vi "Dashboard Main.vi"() -> ()   [LabVIEW 2016]
uses:
  <vilib>/event_ctls.llb/eventvkey.ctl
  <vilib>/Rock Robotics/WPI/Dashboard/WPI_DashboardLogging Global.vi
  <vilib>/Utility/miscctls.llb/LVRowAndColumnTypeDef.ctl
  <vilib>/Rock Robotics/Network Tables/NT Read Numeric Array.vi
  <vilib>/Rock Robotics/Network Tables/NT Read Boolean.vi
panel:
  out "Gear State":string
  in  "Camera Name 2":string(combo)="No Camera Selection"
  in  "Camera Settings Right":T1={"Frame Rate"=30, "Compression"=30, "Size"=1, "DB Camera Config"=FALSE} {"Frame Rate" scale=1.0..30.0; "Compression" scale=100.0..-1.0; "Size" items=["640x480", "320x240", "160x120"]}
  in  "Camera Name Right":string(combo)="No Camera Selection"
  out "Camera Info":cluster{"Mbps LED":bool, "Mbps":dbl, "fps":dbl} {"fps" format="%#.1g"; "Mbps" format="%#.1g"}
  in  "Camera Settings":T1={"Frame Rate"=30, "Compression"=30, "Size"=1, "DB Camera Config"=FALSE} {"Frame Rate" scale=1.0..30.0; "Compression" scale=100.0..-1.0; "Size" items=["640x480", "320x240", "160x120"]}
  in  "TCP":refnum<k5>
  in  "Rec Mode":enum32{"Stop", "Record", "Playback"}(radio)
  out "Robot IP":string
  out "Image Message":string="Timeout in Camera Communications"
  in  "Dashboard Tab":T2(tab)
  in  "Select Auto":string(combo)="Select Autonomous ..."
  out "NT Connection":bool
  out "MotorChart R":cluster{"Numeric":dbl, "Numeric":dbl}(graph)
  out "MotorChart L":cluster{"Numeric":dbl, "Numeric":dbl}(graph)
  out "MotorSliders R":cluster{"MotorSlide1":dbl, "MotorSlide2":dbl} {"MotorSlide2" scale=-1.0..1.0 scale format="%#_2e"; "MotorSlide1" scale=-1.0..1.0 scale format="%#_2e"}
  out "MotorSliders L":cluster{"MotorSlide1":dbl, "MotorSlide2":dbl} {"MotorSlide2" scale=-1.0..1.0 scale format="%#_2e"; "MotorSlide1" scale=-1.0..1.0 scale format="%#_2e"}
  out "Gyro":dbl(knob) scale=0.0..360.0
  out "JS1 Z":dbl(slide) scale=-1.0..1.0 scale format="%#_2e"
  out "JS1 Graph":cluster{"X":dbl, "Y":dbl}[](graph)
  out "JS1 Buttons":T3
  out "JS2 Z":dbl(slide) scale=-1.0..1.0 scale format="%#_2e"
  out "JS2 Graph":cluster{"X":dbl, "Y":dbl}[](graph)
  out "JS2 Buttons":T3
  out "Mode":T4(ring)=enum."Auto Disabled"
  out "Camera Image Right":T5(plugin-control)
  in  "Test Slider":dbl(slide) scale=0.0..100.0 scale format="%#_3g"
  in  "On/Off":bool caption="Solenoid"
  in  "Test Name":u16(ring) items=["Select the test to run..."]
  in  "Test Tree":string(tree)
  in  "Motor":cluster{"Value":dbl, "Enable":bool} {"Value" scale=-1.0..1.0 scale format="%#_3g"}
  out "Progress":T6 {"Test Progress" scale=0.0..100.0}
  in  "Rev/Fwd":cluster{"Forward":bool, "Reverse":bool}
  in  "Test Ring":u16(ring) items=["Monochrome", "Color"]
  out "Cmd Status":string
  in  "Execute Command":bool
  in  "Command Params":string[][](table)
  in  "Command Selection":i32(listbox)
  in  "CheckList":i32(listbox)
  out "Tree":string(tree)
  out "Camera Image":T5(plugin-control)
  out "Background":bool
  in  "Camera Name":string(combo)="No Camera Selection"
  # "HW"
  # "HW"
  # "Joysticks"
  # "Drive Motors"
  # "Front"
  # "Right"
  # "Left"
  # "Back"
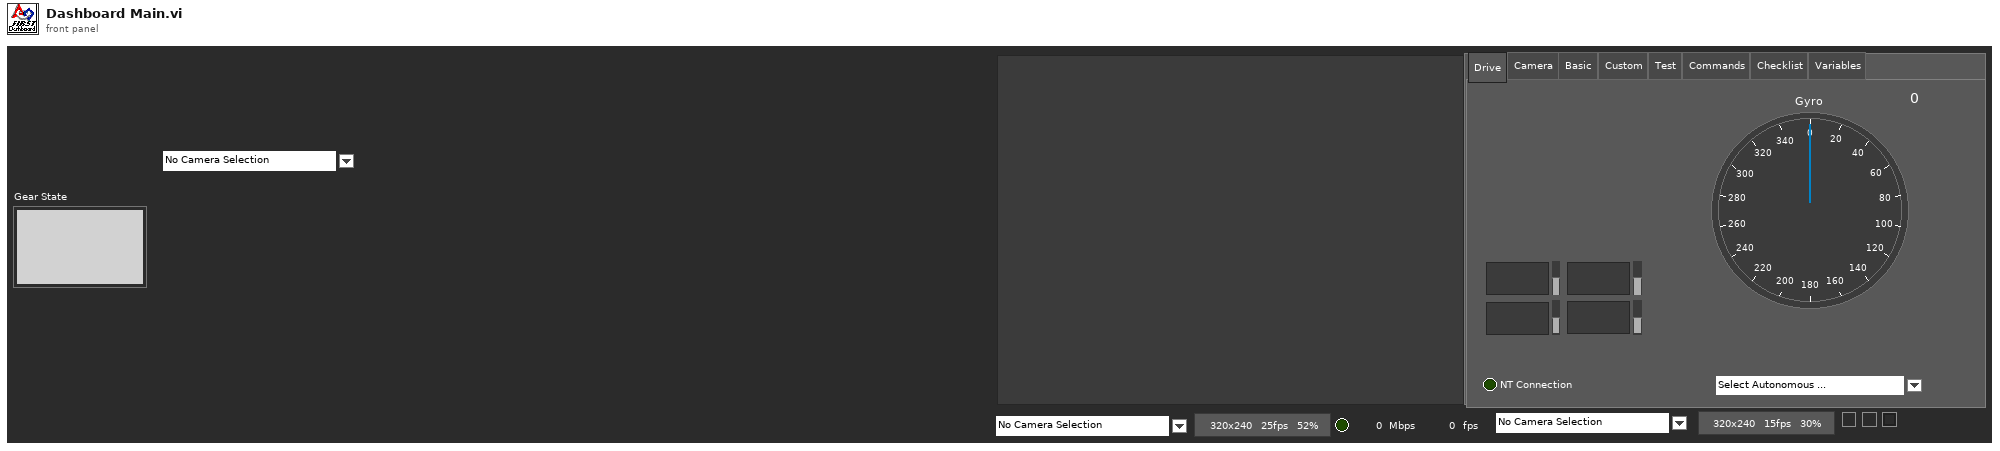
[diagram p1: front panel]
types:
  T1 = cluster{"Frame Rate":i32, "Compression":i32, "Size":u16, "DB Camera Config":bool}
  T2 = enum32{"Drive", "Camera", "Basic", "Custom", "Test", "Commands", "Checklist", "Variables"}
  T3 = cluster{bool, bool, bool, bool, bool, bool, bool, bool, bool, bool, bool, bool}
  T4 = enum8{"Tele-Op Disabled", "Tele-Op Enabled", "Auto Disabled", "Auto Enabled", "Test Disabled", "Test Enabled", "Disconnected", "No Code", "E-Stop"}
  T5 = typedef "IMAQ Image.ctl" = refnum<image>
  T6 = cluster{"Test Progress":u8, "Test Progress Text":string}
  T7 = typedef "Image Type" = u32
  T8 = cluster{"IDs":cluster{"RPC field ID":u16, "Unique ID":u16}, "String":string}
  T9 = enum32{"Drive", "Basic", "Custom", "Test", "Checklist", "Variables"}
  T10 = cluster{"Error Strings":string, "Disable Counts":cluster{u16, u16}, "Rail Faults":cluster{u16, u16, u16}, "Robot IP":string, "DB Mode":u8, "Event Info":cluster{"Name":string, "Type":u8, "Number":u16, "Replay":u8}}
  T11 = cluster{"Storage":cluster{"Disk Free":u64, "RAM Block":u32, "RAM free":u32}, "CPU Utilization":cluster{"CPU % ISR":sgl, "CPU % Time Crit":sgl, "CPU % Timed Str":sgl, "CPU % High":sgl, "CPU % Above":sgl, "CPU % Normal":sgl, "CPU % Low":sgl}, "CAN":cluster{"% Bus Utilization":sgl, "Bus Off Cnt":u32, "TX_FIFO Full Cnt":u32, "Receive Error Cnt":u8, "Transmit Error Cnt":u8}, "HID":cluster{"HID Outputs":u32, "Rumble Low":u16, "Rumble High":u16}[]}
  T12 = cluster{"Status bits":cluster{"Test Mode":bool, "Autonomous":bool, "Enabled":bool, "Code Start":bool, "Brownout":bool, "Reserved 2":bool, "Reserved 3":bool, "E-Stop":bool}, "Code Trace":cluster{"Disabled":bool, "TeleOp":bool, "Auto":bool, "Test":bool}, "Controller Type":enum16{"unknown", "cRIO", "roboRio"}, "Code?":enum16{"unknown", "noCode", "code"}, "Battery V":dbl}
  T13 = cluster{"Control Bits":cluster{"TestMode":bool, "Autonomous":bool, "Enabled":bool, "FMS Present":bool, bool, bool, bool, "E-Stop":bool}, "Team Station ":u8, "Countdown":sgl, "Joystick Values":cluster{"Axes":dbl[], "Buttons":bool[], "POVs":i16[]}[]}
  T14 = cluster{"Axes":dbl[], "Buttons":bool[], "POVs":i16[]}[]
  T15 = cluster{"Axes":dbl[], "Buttons":bool[], "POVs":i16[]}
  T16 = cluster{"Buttons[0]":bool, "Buttons[1]":bool, "Buttons[2]":bool, "Buttons[3]":bool, "Buttons[4]":bool, "Buttons[5]":bool, "Buttons[6]":bool, "Buttons[7]":bool, "Buttons[8]":bool, "Buttons[9]":bool, "Buttons[10]":bool, "Buttons[11]":bool}
  T17 = cluster{"Camera Image":refnum<vi>, "Dashboard Tab":refnum<vi>, "Background":refnum<vi>, "Rec Mode":refnum<vi>, "Test Slider":refnum<vi>, "On/Off ":refnum<vi>, "Test Ring":refnum<vi>, "Rev/Fwd":refnum<vi>, "Test Name":refnum<vi>, "Motor":refnum<vi>, "Progress":refnum<vi>, "CheckList":refnum<vi>, "Tree":refnum<vi>, "Test Tree":refnum<vi>, "Command Params":refnum<vi>, "Command Selection":refnum<vi>, "Execute Command":refnum<vi>, "Cmd Status":refnum<vi>, "Camera Settings":refnum<vi>, "Camera Name":refnum<vi>, "Camera Info":refnum<vi>, "Camera Settings Right":refnum<vi>, "Camera Name Right":refnum<vi>, "Camera Image Right":refnum<vi>}
  T18 = cluster{"Operation":enum16{"Update", "Clear"}, "Color Box":u32}[]
  T19 = typedef "eventvkey.ctl" = enum16{"ASCII", "Enter", "Return", "Shift", "Ctrl", "Alt", "Cmd", "Opt", "Caps", "NumLock", "Clear", "Break", "Up", "Down", "Left", "Right", "Insert", "Delete", "Home", "End", "PageUp", "PageDown", "Escape", "Help", "Pause", "ScrollLock", "F1", "F2", "F3", "F4", "F5", "F6", "F7", "F8", "F9", "F10", "F11", "F12", "F13", "F14", "F15", "F16", "F17", "F18", "F19", "F20", "F21", "F22", "F23", "F24", "Play", "VolumeUp", "VolumeDown", "Mute", "Two Byte Char"}
  T20 = cluster{"Image Size":bool, "Image Type":bool, "Pixel Value":bool, "ROI Information":bool, "Zoom Factor":bool}
  T21 = cluster{"Operation":enum16{"Update", "Clear"}, "Color Box":u32}
  T22 = typedef "LVRowAndColumnTypeDef.ctl" = cluster{"Row":i32, "Column":i32}
  T23 = cluster{"Shift":bool, "Ctrl":bool, "Alt":bool, "Cmd":bool, "Opt":bool}
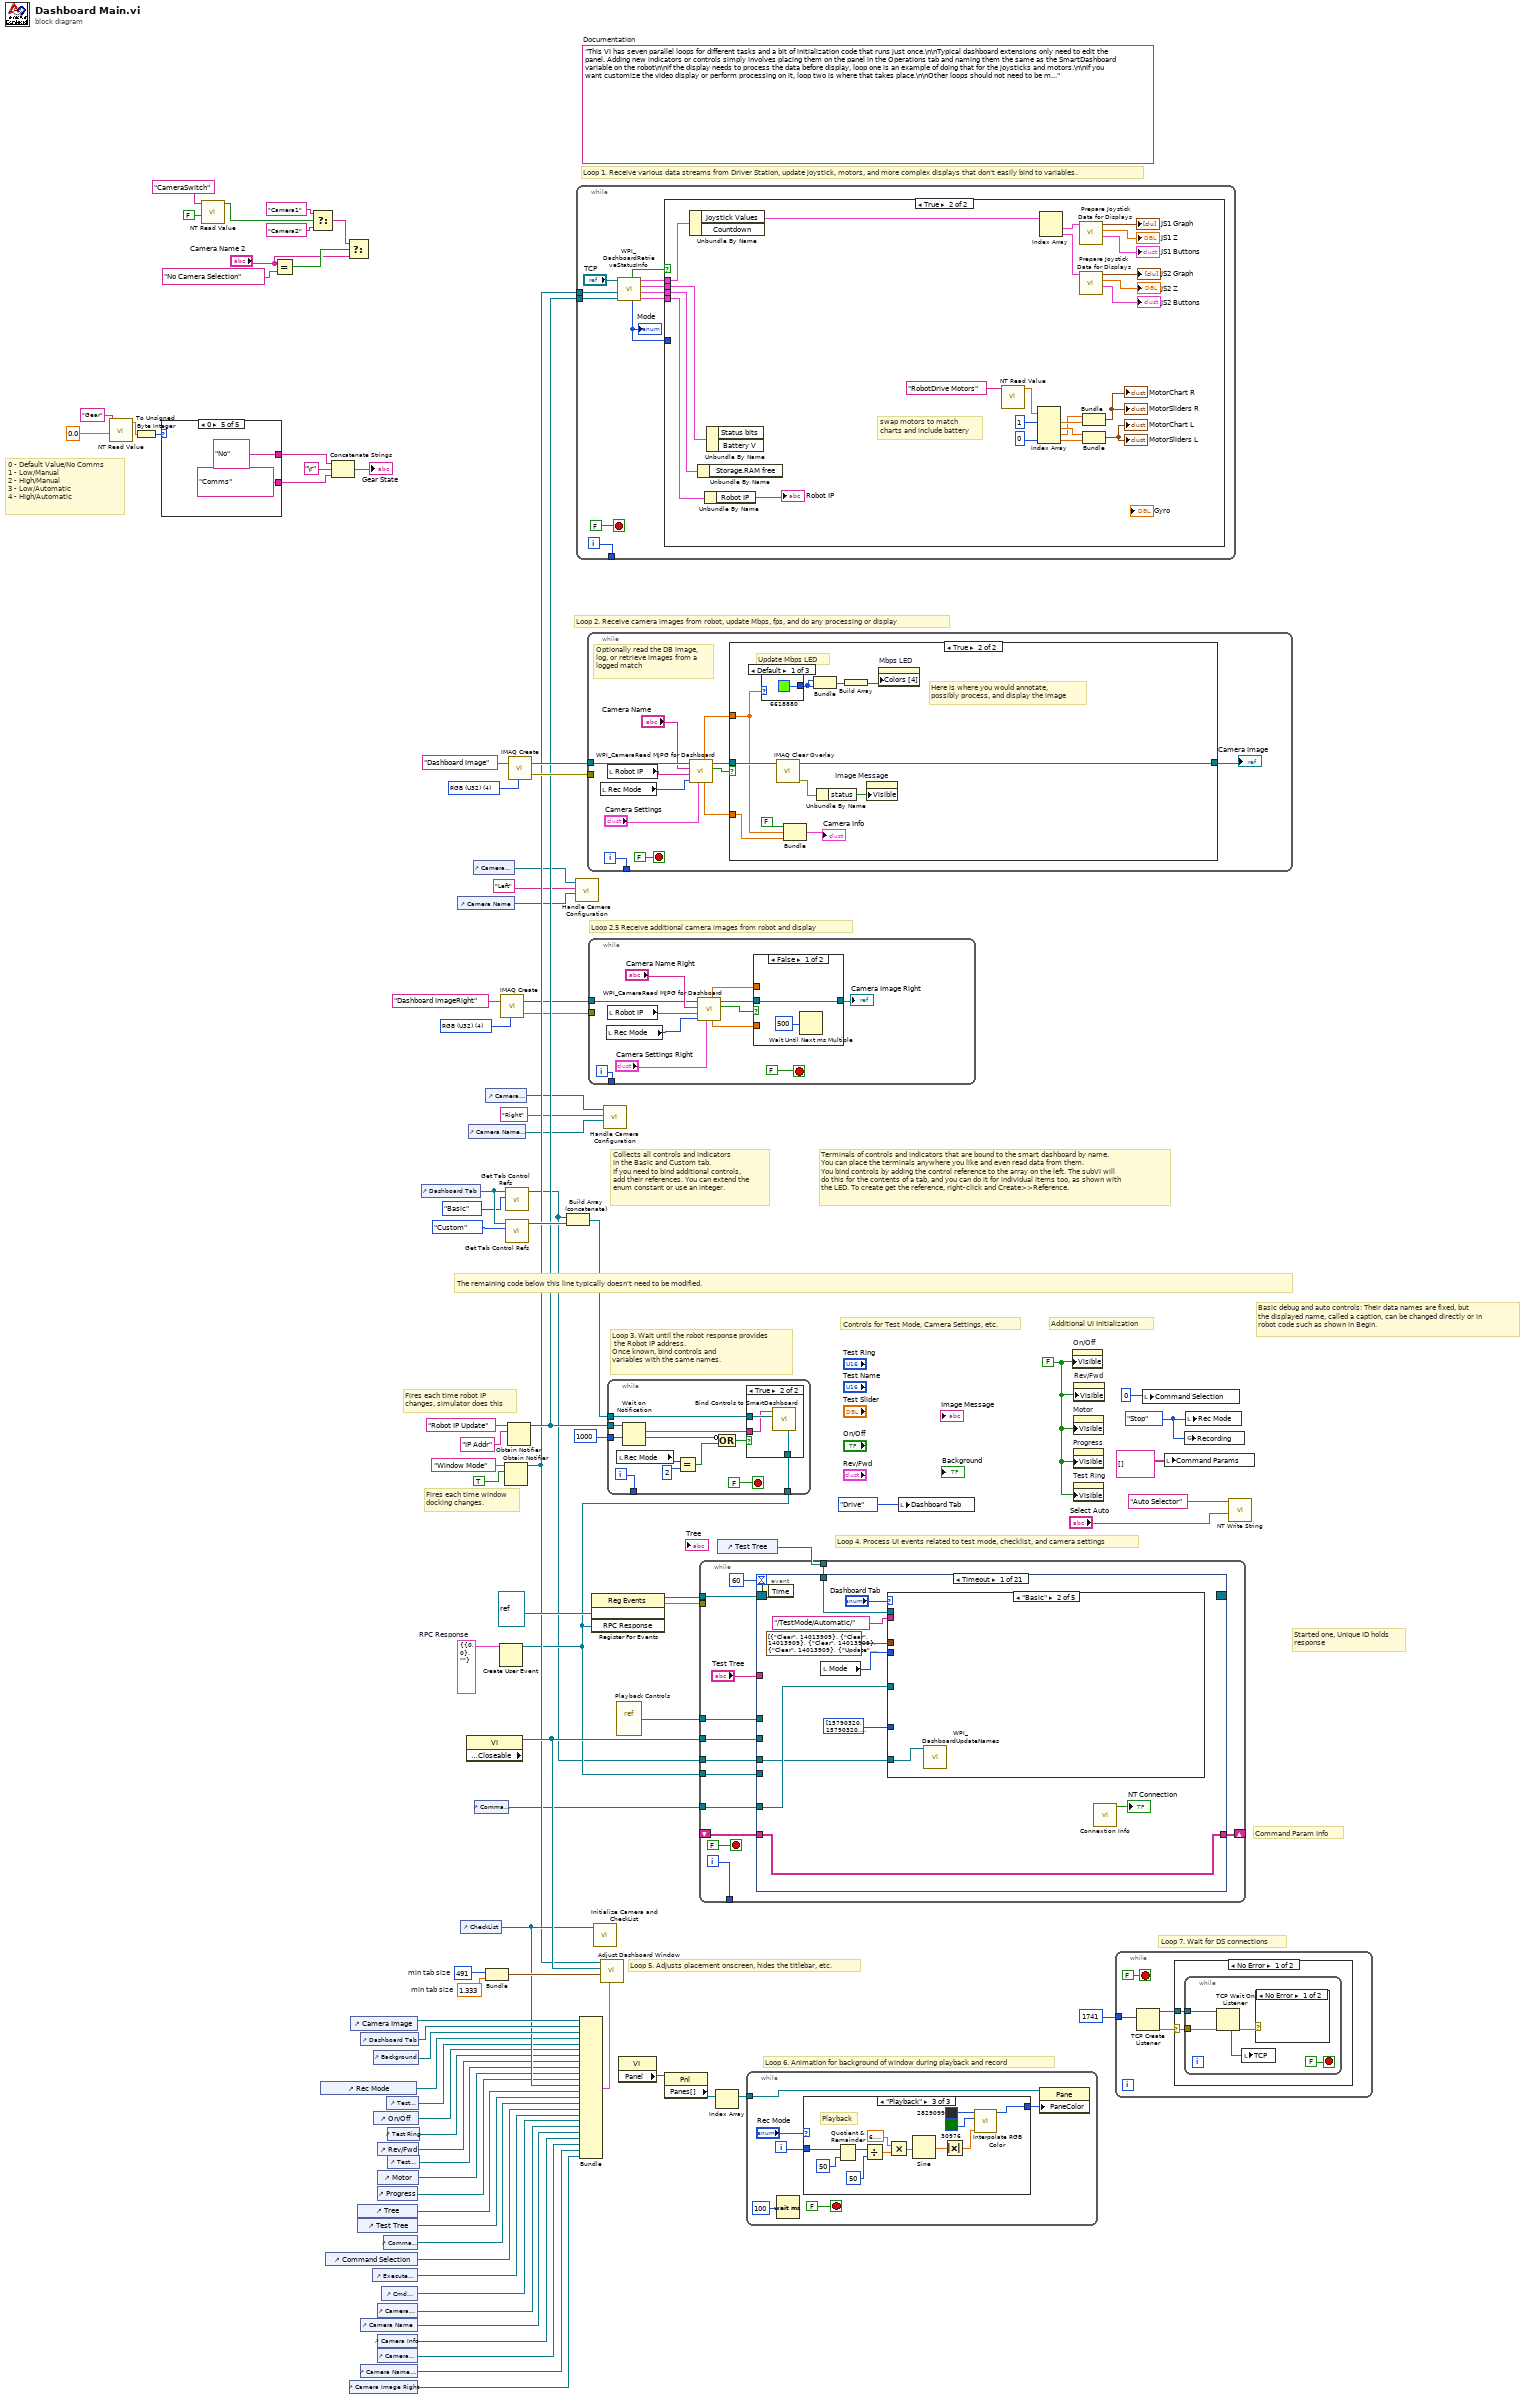
[diagram p0: block diagram]
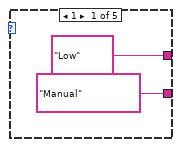
[diagram p2: hidden frame]
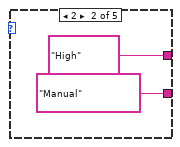
[diagram p3: hidden frame]
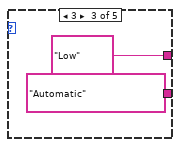
[diagram p4: hidden frame]
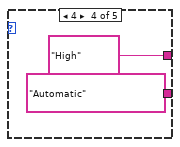
[diagram p5: hidden frame]
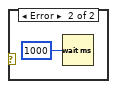
[diagram p7: hidden frame]
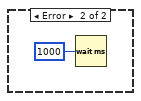
[diagram p8: hidden frame]
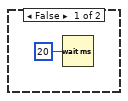
[diagram p9: hidden frame]
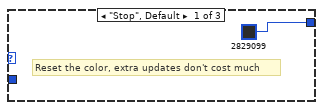
[diagram p10: hidden frame]
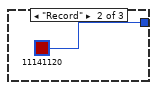
[diagram p11: hidden frame]
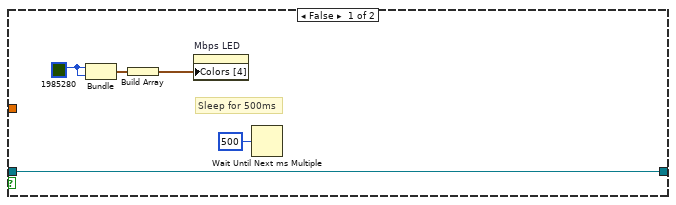
[diagram p13: hidden frame]
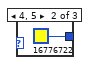
[diagram p14: hidden frame]
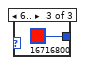
[diagram p15: hidden frame]
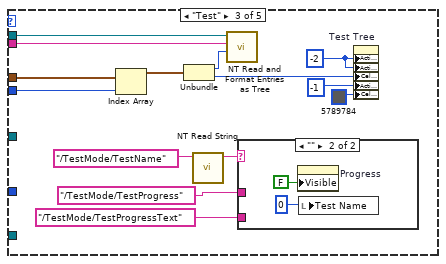
[diagram p17: hidden frame]
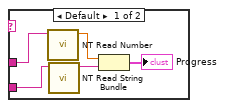
[diagram p18: hidden frame]
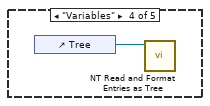
[diagram p19: hidden frame]
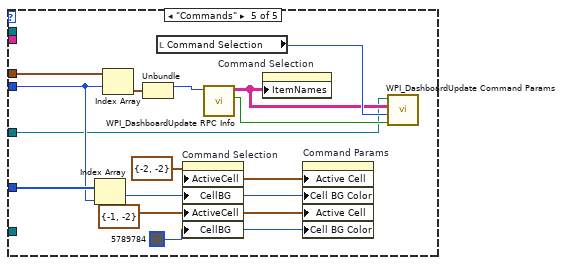
[diagram p20: hidden frame]
diagram:
  w27 = T7 4 items=["Grayscale (U8)", "Grayscale (I16)", "Grayscale (SGL)", "Complex (CSG)", "RGB (U32)", "HSL (U32)", "RGB (U64)"] ("Image Type")
  w43 = T8 {"IDs"={"RPC field ID"=0, "Unique ID"=0}, "String"=""}  # RPC Response
  w68 = 491  # min tab size
  w67 = 1.333  # min tab size
  w75 = enum32{"Stop", "Record", "Playback"}."Stop" ("Rec Mode")
  w50 = FALSE ("Visible")
  (unwired) "This VI has seven parallel loops for different tasks and a bit of initialization code that runs just once.\n\nTypical dashboard extensions only need to edit the panel. Adding new indicators or controls simply involves placing them on the panel in the Operations tab and naming them the same as the SmartDashboard variable on the robot\n\nIf the display needs to process the data before display, loop one is an example of doing that for the joysticks and motors.\n\nIf you want customize the video display or perform processing on it, loop two is where that takes place.\n\nOther loops should not need to be modified. They are pretty standard, and document the task they perform."  # Documentation
  w92 = T7 4 items=["Grayscale (U8)", "Grayscale (I16)", "Grayscale (SGL)", "Complex (CSG)", "RGB (U32)", "HSL (U32)", "RGB (U64)"] ("Image Type")
  # "0 - Default Value/No Comms\n1 - Low/Manual\n2 - High/Manual\n3 - Low/Automatic\n4 - High/Automatic"
  # "Loop 2.5 Receive additional camera images from robot and display"
  # "Command Param Info"
  # "Started one, Unique ID holds\nresponse"
  # "Loop 7. Wait for DS connections"
  # "Basic debug and auto controls: Their data names are fixed, but\nthe displayed name, called a caption, can be changed directly or in\nrobot code such as shown in Begin."
  # "Controls for Test Mode, Camera Settings, etc."
  # "Additional UI Initialization"
  # "Loop 6. Animation for background of window during playback and record"
  # "Fires each time robot IP\nchanges, simulator does this"
  # "Fires each time window\ndocking changes."
  # "Collects all controls and indicators\nin the Basic and Custom tab.\nIf you need to bind additional controls,\nadd their references. You can extend the\nenum constant or use an integer."
  # "The remaining code below this line typically doesn't need to be modified."
  # "Loop 4. Process UI events related to test mode, checklist, and camera settings"
  # "Terminals of controls and indicators that are bound to the smart dashboard by name.\nYou can place the terminals anywhere you like and even read data from them.\nYou bind controls by adding the control reference to the array on the left. The subVI will\ndo this for the contents of a tab, and you can do it for individual items too, as shown with\nthe LED. To create get the reference, right-click and Create>>Reference."
  # "Loop 3. Wait until the robot response provides\n the Robot IP address.\nOnce known, bind controls and\nvariables with the same names."
  # "Loop 5. Adjusts placement onscreen, hides the titlebar, etc."
  # "Loop 1. Receive various data streams from Driver Station, update joystick, motors, and more complex displays that don't easily bind to variables."
  # "Loop 2. Receive camera images from robot, update Mbps, fps, and do any processing or display"
  n1 = call-poly <vilib>:"NT Read Value.vi"("Default Value"=0.0, "Name"="Gear") -> ("Numeric"=w1:dbl)  [unwired: 8 in, 1 out]
  n2 = To Unsigned Byte Integer(number=w1) -> (unsigned 8bit integer=w2:u8)
  n3 = case shown="0" w2 {
    tunnel: ["Low" "High" "Low" "High" "No"] -> w6
    tunnel: ["Manual" "Manual" "Automatic" "Automatic" "Comms"] -> w4
    frame 1 {
    }
    frame 2 {
    }
    frame 3 {
    }
    frame 4 {
    }
    frame 0 {
    }
  }
  n4 = call-poly <vilib>:"NT Read Value.vi"("Default Value"=FALSE, "Name"="CameraSwitch") -> ("Boolean"=w15:bool)  [unwired: 8 in, 1 out]
  n5 = Equal?(x="Camera Name 2", y="No Camera Selection") -> (x = y?=w13:bool)
  n6 = Select(t="Camera1" ("Name"), s=w15, f="Camera2" ("Name")) -> (s? t:f=w12:string)
  n7 = control-ref of="Rec Mode"() -> (w56:refnum<vi>)
  n8 = control-ref of="Command Selection"() -> (w42:refnum<vi>)
  n9 = Concatenate Strings(w6, "\r", w4) -> (→"Gear State":string)
  n10 = Select(t=w12, s=w13, f="Camera Name 2") -> ()  [unwired: 1 out]
  n11 = control-ref of="Camera Image Right"() -> (w18:refnum<vi>)
  n12 = control-ref of="Camera Image"() -> (w70:refnum<vi>)
  n13 = control-ref of="Tree"() -> (w60:refnum<vi>)
  n14 = control-ref of="Test Tree"() -> (w59:refnum<vi>)
  n15 = control-ref of="Dashboard Tab"() -> (w69:refnum<vi>)
  n16 = control-ref of="Camera Name"() -> (w33:refnum<vi>)
  n17 = control-ref of="Camera Name Right"() -> (w19:refnum<vi>)
  n18 = control-ref of="Execute Command"() -> (w44:refnum<vi>)
  n19 = control-ref of="Background"() -> (w65:refnum<vi>)
  n20 = control-ref of="On/Off"() -> (w54:refnum<vi>)
  n21 = control-ref of="Progress"() -> (w51:refnum<vi>)
  n22 = control-ref of="Camera Settings"() -> (w34:refnum<vi>)
  n23 = control-ref of="Camera Info"() -> (w32:refnum<vi>)
  n24 = control-ref of="Camera Settings Right"() -> (w20:refnum<vi>)
  n25 = control-ref of="Rev/Fwd"() -> (w52:refnum<vi>)
  n26 = control-ref of="Motor"() -> (w57:refnum<vi>)
  n27 = control-ref of="Cmd Status"() -> (w38:refnum<vi>)
  n28 = control-ref of="Command Params"() -> (w45:refnum<vi>)
  n29 = control-ref of="Test Slider"() -> (w55:refnum<vi>)
  n30 = control-ref of="Test Ring"() -> (w53:refnum<vi>)
  n31 = control-ref of="Test Name"() -> (w58:refnum<vi>)
  n32 = control-ref of="Dashboard Tab"() -> (w73:refnum<vi>)
  n33 = control-ref of="Camera Name"() -> (w35:refnum<vi>)
  n34 = control-ref of="CheckList"() -> (w61:refnum<vi>)
  n35 = property class="VI" props=["Front Panel.Closeable"]() -> (reference out=w74:refnum<vi>)  [unwired: 2 in, 2 out]
  n36 = control-ref of="Camera Name Right"() -> (w23:refnum<vi>)
  n37 = control-ref of="Camera Settings"() -> (w36:refnum<vi>)
  n38 = control-ref of="Command Params"() -> (w37:refnum<vi>)
  n39 = control-ref of="Camera Settings Right"() -> (w24:refnum<vi>)
  n40 = Bundle("min tab size"=w68, "min tab size"=w67) -> (w66:cluster{"min tab size":i32, "min tab size":dbl})  [unwired: 1 in]
  n41 = Create User Event(user event datatype=w43) -> (user event=w39:refnum<user-event>)  [unwired: 1 in, 1 out]
  n42 = call "IMAQ Create"("Image Name"="Dashboard ImageRight", "Image Type"=w27) -> ("New Image"=w26:T5, "error out"=w25:errorcluster)  [unwired: 2 in, 1 out]
  n43 = Obtain Notifier(name (unnamed)="Window Mode", notification data type=TRUE) -> (notifier out=w48:refnum<notifier>)  [unwired: 2 in, 2 out]
  n44 = call <vilib>:"Get Tab Control Refs.vi"("Page Index"=T9."Basic" ("Dashboard Tab"), "TabControl in"=w73) -> ("ControlsOnPage"=w31:refnum<vi>[])  [unwired: 9 in]
  n45 = call <vilib>:"Get Tab Control Refs.vi"("Page Index"=T9."Custom" ("Dashboard Tab"), "TabControl in"=w73) -> ("ControlsOnPage"=w72:refnum<vi>[])  [unwired: 9 in]
  n46 = Obtain Notifier(name (unnamed)="Robot IP Update", notification data type="IP Addr" ("name (unnamed)")) -> (notifier out=w49:refnum<notifier>)  [unwired: 2 in, 2 out]
  n47 = call "IMAQ Create"("Image Name"="Dashboard Image", "Image Type"=w92) -> ("New Image"=w90:T5, "error out"=w89:errorcluster)  [unwired: 2 in, 1 out]
  n48 = Build Array (concatenate)(w31, w72) -> (w71:refnum<vi>[])
  n49 = call "Handle Camera Configuration.vi"("CameraNameRef"=w35, "Camera File Name"="Left", "ClusterRef"=w36) -> ()  [unwired: 9 in]
  n50 = while {
    tunnel: [w112] -> _
    tunnel: w49 -> [w106]
    tunnel: w48 -> [w103]
    i -> [w112]
    stop <- FALSE stop-if-true
    n51 = call <vilib>:"WPI_DashboardRetrieveStatusInfo.vi"("Binding Refnum"=w106, "Window Mode Notifier"=w103, "TCP Cnx"="TCP") -> ("Power and Errors"=w107:T10, "Robot Metrics"=w110:T11, "Status Info"=w111:T12, "Control Info"=w108:T13, "Robot Mode"=w105:T4, "Process?"=w109:bool)  [unwired: 3 in]
    "Mode" <- w105
    n52 = case shown="True" w109 {
      tunnel: w111 -> [_ w138]
      tunnel: w110 -> [_ w137]
      tunnel: w108 -> [_ w136]
      tunnel: w107 -> [_ w135]
      tunnel: w105 -> [_ _]
      frame False {
        n53 = Wait (ms)(milliseconds to wait=u32 20) -> ()  [unwired: 1 out]
      }
      frame True {
        # "swap motors to match\ncharts and include battery"
        n54 = Unbundle By Name(w136) -> ("Joystick Values"=w126:T14)  [unwired: 1 out]
        n55 = Unbundle By Name(w137) -> ()  [unwired: 1 out]
        n56 = Unbundle By Name(w135) -> ("Robot IP"=→"Robot IP":string)
        n57 = Unbundle By Name(w138) -> ()  [unwired: 2 out]
        n58 = call-poly <vilib>:"NT Read Value.vi"("Name"="RobotDrive Motors") -> ("Numeric Array"=w116:dbl[])  [unwired: 9 in, 1 out]
        n59 = Index Array(array=w116, index #1=1, index #4=0) -> (element #1=w130:dbl, element #2=w131:dbl, element #3=w129:dbl, element #4=w134:dbl)  [unwired: 2 in]
        n60 = Index Array(array=w126) -> (element #1=w125:T15, element #2=w121:T15)  [unwired: 2 in]
        n61 = call "Prepare Joystick Data for Displays.vi"("Joystick Values"=w121) -> ("Buttons"=→"JS2 Buttons":T16, "Z Axis"=→"JS2 Z":dbl, "Cartesian Data"=→"JS2 Graph":cluster{"X axis":dbl, "X axis":dbl}[])  [unwired: 8 in]
        n62 = call "Prepare Joystick Data for Displays.vi"("Joystick Values"=w125) -> ("Buttons"=→"JS1 Buttons":T16, "Z Axis"=→"JS1 Z":dbl, "Cartesian Data"=→"JS1 Graph":cluster{"X axis":dbl, "X axis":dbl}[])  [unwired: 8 in]
        n63 = Bundle("Numeric"=w129, "Numeric"=w130) -> (→"MotorChart R" →"MotorSliders R":cluster{"Numeric":dbl, "Numeric":dbl})  [unwired: 1 in]
        n64 = Bundle("Numeric"=w131, "Numeric"=w134) -> (→"MotorChart L" →"MotorSliders L":cluster{"Numeric":dbl, "Numeric":dbl})  [unwired: 1 in]
      }
    }
  }
  n65 = Bundle("Camera Image"=w70, "Dashboard Tab"=w69, "Background"=w65, "Rec Mode"=w56, "Test Slider"=w55, "On/Off"=w54, "Test Ring"=w53, "Rev/Fwd"=w52, "Test Name"=w58, "Motor"=w57, "Progress"=w51, "CheckList"=w61, "Tree"=w60, "Test Tree"=w59, "Command Params"=w45, "Command Selection"=w42, "Execute Command"=w44, "Cmd Status"=w38, "Camera Settings"=w34, "Camera Name"=w33, "Camera Info"=w32, "Camera Settings Right"=w20, "Camera Name Right"=w19, "Camera Image Right"=w18) -> (w62:T17)  [unwired: 1 in]
  n66 = while {
    tunnel: w90 -> [w148]
    tunnel: w89 -> [_]
    tunnel: [w149] -> _
    i -> [w149]
    stop <- FALSE stop-if-true
    # "Optionally read the DB image,\nlog, or retrieve images from a\nlogged match"
    n67 = local read "Rec Mode"() -> (w144:enum32{"Stop", "Record", "Playback"})
    n68 = local read "Robot IP"() -> (w143:string)
    n69 = call <vilib>:"WPI_CameraRead MJPG for Dashboard.vi"("Camera Settings"="Camera Settings", "Rec Mode"=w144, "Robot IP"=w143, "Camera Name"="Camera Name", "Refnum in"=w148) -> ("Active"=w146:bool, "Refnum out"=w147:T5, "FPS"=w145:dbl, "Bandwidth (Mbps)"=w142:dbl)  [unwired: 3 in]
    n70 = case shown="True" w146 {
      tunnel: w147 -> [w151 w162]
      tunnel: w142 -> [_ w159]
      tunnel: w145 -> [_ w160]
      tunnel: [w151 w156] -> w139
      frame False {
        w153 = u32 1985280 ("Color Box")
        # "Sleep for 500ms"
        n71 = Bundle("Color Box"=w153, "Color Box"=w153) -> (w154:cluster{"Color Box":u32, "Color Box":u32})  [unwired: 1 out]
        n72 = Build Array(w154) -> (w152:cluster{"Color Box":u32, "Color Box":u32}[])
        n73 = property on="Mbps LED" class="Bool (strict)"("Colors [4]"=w152) -> ()  [unwired: 2 in, 2 out]
        n74 = Wait Until Next ms Multiple(millisecond multiple=u32 500) -> ()  [unwired: 1 out]
      }
      frame True {
        # "Here is where you would annotate,\npossibly process, and display the image"
        # "Update Mbps LED"
        n75 = case shown="Default" w159 {
          tunnel: [u32 6618880 ("Color Box") u32 16776722 ("Color Box") u32 16716800 ("Color Box")] -> w163
          frame Default {
          }
          frame 4, 5 {
          }
          frame 6.. {
          }
        }
        n76 = call "IMAQ Clear Overlay"("Image"=w162) -> ("error out"=w165:errorcluster, "Image Out"=w156:T5)  [unwired: 2 in, 7 out]
        n77 = Bundle(FALSE, "Bandwidth (Mbps)"=w159, "FPS"=w160) -> (→"Camera Info":cluster{bool, "Bandwidth (Mbps)":dbl, "FPS":dbl})  [unwired: 1 in]
        n78 = Bundle("Color Box"=w163, "Color Box"=w163) -> (w164:cluster{"Color Box":u32, "Color Box":u32})  [unwired: 1 out]
        n79 = Unbundle By Name(w165) -> ("status"=w166:bool)
        n80 = Build Array(w164) -> (w161:cluster{"Color Box":u32, "Color Box":u32}[])
        n81 = property on="Image Message" class="Str"("Visible"=w166) -> ()  [unwired: 2 in, 2 out]
        n82 = property on="Mbps LED" class="Bool (strict)"("Colors [4]"=w161) -> ()  [unwired: 2 in, 2 out]
      }
    }
    "Camera Image" <- w139
  }
  n83 = while {
    tunnel: w26 -> [w180]
    tunnel: w25 -> [_]
    tunnel: [w174] -> _
    i -> [w174]
    stop <- FALSE stop-if-true
    n84 = local read "Rec Mode"() -> (w178:enum32{"Stop", "Record", "Playback"})
    n85 = local read "Robot IP"() -> (w179:string)
    n86 = call <vilib>:"WPI_CameraRead MJPG for Dashboard.vi"("Camera Settings"="Camera Settings Right", "Rec Mode"=w178, "Robot IP"=w179, "Camera Name"="Camera Name Right", "Refnum in"=w180) -> ("Active"=w173:bool, "Refnum out"=w176:T5, "FPS"=w171:dbl, "Bandwidth (Mbps)"=w172:dbl)  [unwired: 3 in]
    n87 = case shown="False" w173 {
      tunnel: w176 -> [w182 w184]
      tunnel: w172 -> [_ _]
      tunnel: w171 -> [_ _]
      tunnel: [w182 w184] -> w170
      frame False {
        n88 = Wait Until Next ms Multiple(millisecond multiple=u32 500) -> ()  [unwired: 1 out]
      }
      frame True {
      }
    }
    "Camera Image Right" <- w170
  }
  n89 = register-events(refnum<vi> refnum, w39) -> (reference out=w79:refnum<event-registration>, error out=w78:errorcluster)  [unwired: 2 in]
  n90 = call "Initialize Camera and CheckList.vi"("ListBox in"=w61) -> ()  [unwired: 11 in]
  n91 = call "Adjust Dashboard Window.vi"("Sizing Refnums"=w62, "Size Constraints"=w66, "VI"=w74, "WIn Mode"=w48) -> ()  [unwired: 8 in]
  n92 = call "Handle Camera Configuration.vi"("CameraNameRef"=w23, "Camera File Name"="Right", "ClusterRef"=w24) -> ()  [unwired: 9 in]
  n93 = while {
    tunnel: w71 -> [w196]
    tunnel: w49 -> [w194]
    tunnel: [w192] -> _
    tunnel: u32 1000 ("milliseconds to wait") -> [w191]
    tunnel: w39 -> [w185]
    i -> [w192]
    stop <- FALSE stop-if-true
    n94 = local read "Rec Mode"() -> (w187:enum32{"Stop", "Record", "Playback"})
    n95 = Wait on Notification(notifier=w194, timeout in ms (-1)=w191) -> (notification=w193:string, timed out?=w189:bool)  [unwired: 2 in, 2 out]
    n96 = Equal?(x=w187, y=u16 2 ("Rec Mode")) -> (x = y?=w188:bool)
    n97 = Compound Arithmetic op=OR(invert w189, w188) -> (w190:bool)
    n98 = case shown="True" w190 {
      tunnel: w196 -> [_ w199]
      tunnel: w193 -> [_ w198]
      tunnel: w185 -> [_ w197]
      frame False {
      }
      frame True {
        n99 = call <vilib>:"Bind Controls to SmartDashboard.vi"("RPC ref"=w197, "Bound Control Refs"=w199, "Server IP Address"=w198) -> ()  [unwired: 9 in]
      }
    }
  }
  n100 = vi-ref "Playback Controls.vi"() -> (w80:refnum<vi>)
  n101 = property class="VI"() -> ("Panel"=w82:refnum<vi>)  [unwired: 2 in, 2 out]
  n102 = property class="Pnl"(reference=w82) -> ("Panes[]"=w83:refnum<vi>[])  [unwired: 1 in, 2 out]
  n103 = Index Array(array=w83) -> (element=w81:refnum<vi>)  [unwired: 1 in]
  n104 = control-ref of="Test Tree"() -> (w84:refnum<vi>)
  n105 = while {
    tunnel: [w209] -> _
    tunnel: w84 -> [w208]
    tunnel: w80 -> [w207]
    tunnel: w79 -> [w206]
    tunnel: w78 -> [_]
    tunnel: w74 -> [w205]
    tunnel: w39 -> [w204]
    tunnel: w37 -> [w203]
    shift-right: [w202] -> _
    shift-left: _ -> [w201]
    tunnel: w31 -> [w200]
    i -> [w209]
    stop <- FALSE stop-if-true
    n106 = event shown="[0] Timeout" {
      selector: w206 -> [_ _ _ _ _ _ _ _ _ _ _ _ _ _ _ _ _ _ _ _ _]
      dyn-events: [_ _ _ _ _ _ _ _ _ _ _ _ _ _ _ _ w465 _ _ _ _] -> _
      timeout: u32 60 ("milliseconds to wait") -> [_ _ _ _ _ _ _ _ _ _ _ _ _ _ _ _ _ _ _ _ _]
      tunnel: w208 -> [w221 _ _ _ _ _ _ _ _ _ _ _ _ _ _ _ _ _ _ _ _]
      tunnel: "Test Tree" -> [_ _ _ _ _ _ _ _ _ _ _ w432 w440 w442 w446 w454 _ _ _ _ _]
      tunnel: w207 -> [_ _ _ _ _ _ _ _ _ _ _ _ _ _ _ _ w467 _ w485 _ _]
      tunnel: w205 -> [_ _ _ _ _ _ _ _ _ _ _ _ _ _ _ _ w463 _ _ _ _]
      tunnel: w204 -> [_ _ _ _ _ _ _ _ _ _ _ _ _ _ _ _ w459 _ _ _ _]
      tunnel: w203 -> [w216 _ _ _ _ _ w383 _ _ _ _ _ _ _ _ _ _ _ _ _ _]
      tunnel: [w215 w260 w362 w367 w376 w380 w381 w390 w400 w407 w419 w431 w438 w441 w445 w453 w458 w480 w482 w486 w497] -> w202
      tunnel: w201 -> [w215 w260 w362 w367 w376 w380 w381 _ _ w407 w419 w431 w438 w441 w445 w453 w458 w480 w482 w486 w497]
      tunnel: w200 -> [w213 _ _ _ _ _ _ _ _ _ _ _ _ _ _ _ _ _ _ _ _]
      event Timeout {
        n107 = event-data() -> ()  [unwired: 1 in, 1 out]
        n108 = local read "Mode"() -> (w218:T4)
        n109 = case shown="\"Basic\"" "Dashboard Tab" {
          tunnel: w221 -> [_ _ w237 _ _]
          tunnel: "/TestMode/Automatic/" ("Name Pattern") -> [_ _ w236 _ _]
          tunnel: T18 [{"Operation"=enum."Clear", "Color Box"=14013909}, {"Operation"=enum."Clear", "Color Box"=14013909}, {"Operation"=enum."Clear", "Color Box"=14013909}, {"Operation"=enum."Clear", "Color Box"=14013909}, {"Operation"=enum."Update", "Color Box"=14013909}, {"Operation"=enum."Update", "Color Box"=16777215}, {"Operation"=enum."Clear", "Color Box"=14013909}, {"Operation"=enum."Clear", "Color Box"=14013909}, {"Operation"=enum."Clear", "Color Box"=14013909}] -> [_ _ w229 _ w253]
          tunnel: w218 -> [_ _ w228 _ w252]
          tunnel: u32[] [15790320, 15790320, 15790320, 15790320, 16777215, 16777215, 15790320, 15790320, 15790320] -> [_ _ _ _ w258]
          tunnel: w216 -> [_ _ _ _ w246]
          tunnel: w213 -> [_ w223 _ _ _]
          frame "Custom", Default {
          }
          frame "Basic" {
            n110 = call <vilib>:"WPI_DashboardUpdateNames.vi"("Controls on Tab"=w223) -> ()  [unwired: 11 in]
          }
          frame "Test" {
            w235 = -2 ("Active Item:Row Number")
            n111 = Index Array(array=w229, index=w228) -> (element=w230:T21)
            n112 = Unbundle(w230) -> ("Operation"=w231:enum16{"Update", "Clear"}, "Color Box"=w232:u32)
            n113 = call <vilib>:"NT Read String.vi"("Name"="/TestMode/TestName") -> ("String"=w226:string)  [unwired: 9 in, 1 out]
            n114 = call <vilib>:"NT Read and Format Entries as Tree.vi"("Operation"=w231, "Name Pattern"=w236, "Tree Refnum"=w237) -> ()  [unwired: 7 in, 2 out]
            n115 = case shown="\"\"" w226 {
              tunnel: "/TestMode/TestProgress" ("Name") -> [w239 _]
              tunnel: "/TestMode/TestProgressText" ("Name") -> [w238 _]
              frame Default {
                n116 = call <vilib>:"NT Read Number.vi"("Name"=w239) -> ("Numeric"=w240:dbl)  [unwired: 9 in, 1 out]
                n117 = call <vilib>:"NT Read String.vi"("Name"=w238) -> ("String"=w241:string)  [unwired: 9 in, 1 out]
                n118 = Bundle("Numeric"=w240, "String"=w241) -> (→"Progress":cluster{"Numeric":dbl, "String":string})  [unwired: 1 in]
              }
              frame "" {
                n119 = property on="Progress" class="Clust (strict)"("Visible"=FALSE) -> ()  [unwired: 2 in, 2 out]
                n120 = local write "Test Name"(u16 0) -> ()
              }
            }
            n121 = property on="Test Tree" class="Tree (strict)"("Active Item Row Number"=w235, "ActiveColNum"=w235, "CellBG"=w232, "Active Item Row Number"=-1 ("Active Item:Row Number"), "CellBG"=u32 5789784 ("Color Box")) -> ()  [unwired: 2 in, 2 out]
          }
          frame "Variables" {
            n122 = control-ref of="Tree"() -> (w245:refnum<vi>)
            n123 = call <vilib>:"NT Read and Format Entries as Tree.vi"("Tree Refnum"=w245) -> ()  [unwired: 9 in, 2 out]
          }
          frame "Commands" {
            w254 = u32 5789784 ("Color Box")
            w255 = T22 {"Row"=-1, "Column"=-2} ("Active Cell:Active Cell")
            w257 = T22 {"Row"=-2, "Column"=-2} ("Active Cell:Active Cell")
            n124 = Index Array(array=w258, index=w252) -> (element=w256:u32)
            n125 = Index Array(array=w253, index=w252) -> (element=w251:T21)
            n126 = Unbundle(w251) -> ("Operation"=w250:enum16{"Update", "Clear"})  [unwired: 1 out]
            n127 = local read "Command Selection"() -> (w249:i32)
            n128 = property on="Command Selection" class="MCListbox (strict)"("ActiveCell"=w257, "CellBG"=w256, "ActiveCell"=w255, "CellBG"=w254) -> ()  [unwired: 2 in, 2 out]
            n129 = call <vilib>:"WPI_DashboardUpdate RPC Info.vi"("Operation"=w250) -> ("update"=w248:bool, "commands"=w247:string[][])  [unwired: 9 in]
            n130 = property on="Command Selection" class="MCListbox (strict)"("ItemNames"=w247) -> ()  [unwired: 2 in, 2 out]
            n131 = property on="Command Params" class="Tbl (strict)"("Active Cell"=w257, "Cell BG Color"=w256, "Active Cell"=w255, "Cell BG Color"=w254) -> ()  [unwired: 2 in, 2 out]
            n132 = call <vilib>:"WPI_DashboardUpdate Command Params.vi"("Update"=w248, "NewVal"=w249, "Commands"=w247, "Param Tbl"=w246) -> ()  [unwired: 7 in, 1 out]
          }
        }
        n133 = call <vilib>:"Connextion Info.vi"() -> ("Connected"=→"NT Connection":bool)  [unwired: 10 in, 1 out]
      }
      event "Test Tree": Value Change {
        # "Show appropriate\ncontrols"
        n134 = event-data() -> ("CtlRef"=w263:refnum<vi>, "NewVal"=w261:string)  [unwired: 1 in]
        n135 = call <vilib>:"WPI_UtilitiesGetTreeIOName.vi"("NewVal"=w261, "TreeControl in"=w263) -> ("I/O Name"=w264:string)  [unwired: 9 in]
        n136 = case shown="\"Camera\"" w264 {
          selector: w264 -> [_ w271 _ w293 w302 _]
          tunnel: w261 -> [_ _ w290 w292 _ w309]
          tunnel: cluster{string[]}[] [{["640x480", "320x240", "160x120"]}, {["Auto", "Fixed indoor", "Fixed outdoor 1", "Fixed outdoor 2", "Fixed fluorescent 1", "Fixed fluorescent 2", "Hold current"]}, {["Auto", "Flicker-free 50 Hz", "Flicker-free 60 Hz", "Hold current"]}, {["None", "Prioritize frame rate", "Prioritize image quality"]}, {["Monochrome", "Color"]}] -> [_ _ _ _ _ w308]
          frame Default {
            w266 = FALSE ("Visible")
            w265 = FALSE ("Visible")
            n137 = property on="Motor" class="Clust (strict)"("Visible"=w265) -> ()  [unwired: 2 in, 2 out]
            n138 = property on="Test Ring" class="Ring (strict)"("Visible"=w265) -> ()  [unwired: 2 in, 2 out]
            n139 = property on="Rev/Fwd" class="Clust (strict)"("Visible"=w266) -> ()  [unwired: 2 in, 2 out]
            n140 = property on="On/Off" class="Bool (strict)"("Visible"=w266) -> ()  [unwired: 2 in, 2 out]
            n141 = property on="Test Slider" class="Slide (strict)"("Visible"=w266) -> ()  [unwired: 2 in, 2 out]
          }
          frame "Analog Out", "Motor", "PWM" {
            w272 = FALSE ("Visible")
            n142 = case shown="\"Analog Out\"" w271 {
              tunnel: [1.0 ("Value") -1.0 ("Value") 0.0 ("Value")] -> w270
              tunnel: [255.0 ("Value") 1.0 ("Value") 5.0 ("Value")] -> w269
              tunnel: [128.0 ("Value") 0.0 ("Value") 0.0 ("Value")] -> w268
              tunnel: [64.0 ("Value") 0.5 ("Value") 1.0 ("Value")] -> w267
              frame "PWM" {
              }
              frame "Motor", Default {
              }
              frame "Analog Out" {
              }
            }
            n143 = property on="Motor" class="Clust (strict)"("Visible"=TRUE) -> ()  [unwired: 2 in, 2 out]
            n144 = property on="Value" class="Slide (strict)"("Value"=w268, "Scale.Minimum"=w270, "Scale.Maximum"=w269, "Scale.Increment"=w267) -> ()  [unwired: 2 in, 2 out]
            n145 = property on="On/Off" class="Bool (strict)"("Visible"=w272) -> ()  [unwired: 2 in, 2 out]
            n146 = property on="Test Slider" class="Slide (strict)"("Visible"=w272) -> ()  [unwired: 2 in, 2 out]
            n147 = property on="Test Ring" class="Ring (strict)"("Visible"=w272) -> ()  [unwired: 2 in, 2 out]
            n148 = property on="Rev/Fwd" class="Clust (strict)"("Visible"=w272) -> ()  [unwired: 2 in, 2 out]
          }
          frame "Servo" {
            w288 = FALSE ("Visible")
            n149 = call <vilib>:"NT Read Number.vi"("Name"=w290) -> ("Numeric"=w289:dbl)  [unwired: 9 in, 1 out]
            n150 = property on="Test Slider" class="Slide (strict)"("Visible"=TRUE, "Scale.Maximum"=170.0 ("Scale.Range:Maximum")) -> ()  [unwired: 2 in, 2 out]
            n151 = local write "Test Slider"(w289) -> ()
            n152 = property on="Motor" class="Clust (strict)"("Visible"=w288) -> ()  [unwired: 2 in, 2 out]
            n153 = property on="Rev/Fwd" class="Clust (strict)"("Visible"=w288) -> ()  [unwired: 2 in, 2 out]
            n154 = property on="On/Off" class="Bool (strict)"("Visible"=w288) -> ()  [unwired: 2 in, 2 out]
            n155 = property on="Test Ring" class="Ring (strict)"("Visible"=w288) -> ()  [unwired: 2 in, 2 out]
          }
          frame "Relay", "Solenoid" {
            w291 = FALSE ("Visible")
            n156 = property on="Motor" class="Clust (strict)"("Visible"=w291) -> ()  [unwired: 2 in, 2 out]
            n157 = property on="Test Slider" class="Slide (strict)"("Visible"=w291) -> ()  [unwired: 2 in, 2 out]
            n158 = Search and Replace String(input string=w292, search string="/Value  **", replace string="/Direction") -> (result string=w298:string)  [unwired: 5 in, 3 out]
            n159 = property on="Test Ring" class="Ring (strict)"("Visible"=w291) -> ()  [unwired: 2 in, 2 out]
            n160 = call <vilib>:"NT Read String.vi"("Name"=w298) -> ("String"=w296:string)  [unwired: 9 in, 1 out]
            n161 = Equal?(x="Both directions", y=w296) -> (x = y?=w294:bool)
            n162 = Not(x=w294) -> (.not. x?=w295:bool)
            n163 = property on="Rev/Fwd" class="Clust (strict)"("Visible"=w294) -> ()  [unwired: 2 in, 2 out]
            n164 = property on="On/Off" class="Bool (strict)"("Visible"=w295, "Caption.Text"=w293) -> ()  [unwired: 2 in, 2 out]
          }
          frame "Compressor", "Digital Out" {
            w301 = FALSE ("Visible")
            # "Get direction and finish"
            n165 = property on="Motor" class="Clust (strict)"("Visible"=w301) -> ()  [unwired: 2 in, 2 out]
            n166 = property on="Test Slider" class="Slide (strict)"("Visible"=w301) -> ()  [unwired: 2 in, 2 out]
            n167 = property on="Test Ring" class="Ring (strict)"("Visible"=w301) -> ()  [unwired: 2 in, 2 out]
            n168 = property on="On/Off" class="Bool (strict)"("Visible"=TRUE, "Caption.Text"=w302) -> ()  [unwired: 2 in, 2 out]
            n169 = property on="Rev/Fwd" class="Clust (strict)"("Visible"=FALSE) -> ()  [unwired: 2 in, 2 out]
          }
          frame "Camera" {
            n170 = call <vilib>:"Get Last Path Segment.vi"("String in"=w309) -> ("String out"=w310:string)  [unwired: 10 in]
            n171 = property on="On/Off" class="Bool (strict)"("Visible"=FALSE) -> ()  [unwired: 2 in, 2 out]
            n172 = property on="Motor" class="Clust (strict)"("Visible"=FALSE) -> ()  [unwired: 2 in, 2 out]
            n173 = property on="Rev/Fwd" class="Clust (strict)"("Visible"=FALSE) -> ()  [unwired: 2 in, 2 out]
            n174 = case shown="\"White Balance  **\"" w310 {
              tunnel: w309 -> [w316 w325 w334 w343 w352 _ w358]
              tunnel: w308 -> [w314 w322 w331 w340 w349 _ _]
              frame "Size  **" {
                n175 = Index Array(array=w314) -> (element=w313:cluster{string[]})  [unwired: 1 in]
                n176 = call <vilib>:"NT Read String.vi"("Name"=w316) -> ("String"=w315:string)  [unwired: 9 in, 1 out]
                n177 = Unbundle(w313) -> (w311:string[])
                n178 = Match First String(2:w311, 3:w315) -> (0:w312:i32)  [unwired: 1 out]
                n179 = property on="Test Ring" class="Ring (strict)"("Value"=w312, "Strings []"=w311) -> ()  [unwired: 2 in, 2 out]
                n180 = property on="Test Ring" class="Ring (strict)"("Visible"=TRUE) -> ()  [unwired: 2 in, 2 out]
                n181 = property on="Test Slider" class="Slide (strict)"("Visible"=FALSE) -> ()  [unwired: 2 in, 2 out]
              }
              frame "White Balance  **" {
                n182 = Index Array(array=w322, index=1) -> (element=w323:cluster{string[]})
                n183 = call <vilib>:"NT Read String.vi"("Name"=w325) -> ("String"=w324:string)  [unwired: 9 in, 1 out]
                n184 = Unbundle(w323) -> (w320:string[])
                n185 = Match First String(2:w320, 3:w324) -> (0:w319:i32)  [unwired: 1 out]
                n186 = property on="Test Ring" class="Ring (strict)"("Value"=w319, "Strings []"=w320) -> ()  [unwired: 2 in, 2 out]
                n187 = property on="Test Ring" class="Ring (strict)"("Visible"=TRUE) -> ()  [unwired: 2 in, 2 out]
                n188 = property on="Test Slider" class="Slide (strict)"("Visible"=FALSE) -> ()  [unwired: 2 in, 2 out]
              }
              frame "Exposure  **" {
                n189 = Index Array(array=w331, index=2) -> (element=w332:cluster{string[]})
                n190 = call <vilib>:"NT Read String.vi"("Name"=w334) -> ("String"=w333:string)  [unwired: 9 in, 1 out]
                n191 = Unbundle(w332) -> (w328:string[])
                n192 = Match First String(2:w328, 3:w333) -> (0:w329:i32)  [unwired: 1 out]
                n193 = property on="Test Ring" class="Ring (strict)"("Value"=w329, "Strings []"=w328) -> ()  [unwired: 2 in, 2 out]
                n194 = property on="Test Ring" class="Ring (strict)"("Visible"=TRUE) -> ()  [unwired: 2 in, 2 out]
                n195 = property on="Test Slider" class="Slide (strict)"("Visible"=FALSE) -> ()  [unwired: 2 in, 2 out]
              }
              frame "Exposure Priority  **" {
                n196 = Index Array(array=w340, index=3) -> (element=w341:cluster{string[]})
                n197 = call <vilib>:"NT Read String.vi"("Name"=w343) -> ("String"=w342:string)  [unwired: 9 in, 1 out]
                n198 = Unbundle(w341) -> (w337:string[])
                n199 = Match First String(2:w337, 3:w342) -> (0:w338:i32)  [unwired: 1 out]
                n200 = property on="Test Ring" class="Ring (strict)"("Value"=w338, "Strings []"=w337) -> ()  [unwired: 2 in, 2 out]
                n201 = property on="Test Ring" class="Ring (strict)"("Visible"=TRUE) -> ()  [unwired: 2 in, 2 out]
                n202 = property on="Test Slider" class="Slide (strict)"("Visible"=FALSE) -> ()  [unwired: 2 in, 2 out]
              }
              frame "Color Enable  **" {
                n203 = Index Array(array=w349, index=4) -> (element=w350:cluster{string[]})
                n204 = call <vilib>:"NT Read String.vi"("Name"=w352) -> ("String"=w351:string)  [unwired: 9 in, 1 out]
                n205 = Unbundle(w350) -> (w346:string[])
                n206 = Match First String(2:w346, 3:w351) -> (0:w347:i32)  [unwired: 1 out]
                n207 = property on="Test Ring" class="Ring (strict)"("Value"=w347, "Strings []"=w346) -> ()  [unwired: 2 in, 2 out]
                n208 = property on="Test Ring" class="Ring (strict)"("Visible"=TRUE) -> ()  [unwired: 2 in, 2 out]
                n209 = property on="Test Slider" class="Slide (strict)"("Visible"=FALSE) -> ()  [unwired: 2 in, 2 out]
              }
              frame Default {
                n210 = property on="Test Ring" class="Ring (strict)"("Visible"=FALSE) -> ()  [unwired: 2 in, 2 out]
                n211 = property on="Test Slider" class="Slide (strict)"("Visible"=FALSE) -> ()  [unwired: 2 in, 2 out]
              }
              frame "Brightness  **", "Color Level  **", "Compression  **", "FPS  **", "Sharpness  **" {
                n212 = call <vilib>:"NT Read Number.vi"("Name"=w358) -> ("Numeric"=w357:dbl)  [unwired: 9 in, 1 out]
                n213 = local write "Test Slider"(w357) -> ()
                n214 = property on="Test Slider" class="Slide (strict)"("Visible"=TRUE, "Scale.Maximum"=100.0 ("Scale.Range:Maximum")) -> ()  [unwired: 2 in, 2 out]
                n215 = property on="Test Ring" class="Ring (strict)"("Visible"=FALSE) -> ()  [unwired: 2 in, 2 out]
              }
            }
          }
        }
        n216 = property on="Progress" class="Clust (strict)"("Visible"=FALSE) -> ()  [unwired: 2 in, 2 out]
      }
      event "Test Name": Mouse Enter {
        # "Populate the ring with the list of tests"
        n217 = event-data() -> ()  [unwired: 1 in, 1 out]
        n218 = call <vilib>:"NT Read String Array.vi"("Name"="/TestMode/TestList") -> ("String Array"=w366:string[])  [unwired: 9 in, 1 out]
        n219 = Build Array (concatenate)("Select the test to run...", w366) -> (w365:string[])
        n220 = property on="Test Name" class="Ring (strict)"("Strings []"=w365) -> ()  [unwired: 2 in, 2 out]
      }
      event "Test Name": Value Change {
        w368 = FALSE ("Visible")
        # "Tell the robot the test name to run"
        n221 = event-data() -> ("NewVal"=w372:u16)  [unwired: 1 in]
        n222 = property on="Test Name" class="Ring (strict)"() -> ("Strings []"=w373:string[])  [unwired: 2 in, 2 out]
        n223 = local write "Progress"(T6 {"Test Progress"=0, "Test Progress Text"=""} ("Progress")) -> ()
        n224 = Index Array(array=w373, index=w372) -> (element=w371:string)
        n225 = call <vilib>:"NT Write String.vi"("String"=w371, "Name"="/TestMode/TestName") -> ()  [unwired: 9 in, 1 out]
        n226 = property on="Progress" class="Clust (strict)"("Visible"=TRUE) -> ()  [unwired: 2 in, 2 out]
        n227 = property on="Motor" class="Clust (strict)"("Visible"=w368) -> ()  [unwired: 2 in, 2 out]
        n228 = property on="Test Slider" class="Slide (strict)"("Visible"=w368) -> ()  [unwired: 2 in, 2 out]
        n229 = property on="On/Off" class="Bool (strict)"("Visible"=w368) -> ()  [unwired: 2 in, 2 out]
        n230 = property on="Rev/Fwd" class="Clust (strict)"("Visible"=w368) -> ()  [unwired: 2 in, 2 out]
        n231 = property on="Test Ring" class="Ring (strict)"("Visible"=w368) -> ()  [unwired: 2 in, 2 out]
      }
      event "Select Auto": Mouse Enter {
        # "Populate the combo box with the list of autonomous options"
        n232 = event-data() -> ()  [unwired: 1 in, 1 out]
        n233 = call <vilib>:"NT Read String Array.vi"("Name"="Auto List") -> ("String Array"=w375:string[])  [unwired: 9 in, 1 out]
        n234 = property on="Select Auto" class="CmbBox"("Strings[]"=w375) -> ()  [unwired: 2 in, 2 out]
      }
      event "Select Auto": Value Change {
        # "User modified the Auto Selection. Write to NT variable so robot knows."
        n235 = event-data() -> ("NewVal"=w378:string)  [unwired: 1 in]
        n236 = call <vilib>:"NT Write String.vi"("String"=w378, "Name"="Auto Selector") -> ()  [unwired: 9 in, 1 out]
      }
      event "Command Selection": Value Change {
        # "Get the params and show in table"
        n237 = event-data() -> ("NewVal"=w384:i32)  [unwired: 1 in]
        n238 = property on="Command Selection" class="MCListbox (strict)"() -> ("ItemNames"=w382:string[][])  [unwired: 2 in, 2 out]
        n239 = call <vilib>:"WPI_DashboardUpdate Command Params.vi"("NewVal"=w384, "Commands"=w382, "Param Tbl"=w383) -> ()  [unwired: 8 in, 1 out]
      }
      event "Execute Command": Value Change {
        # "Started one, Unique ID holds\nresponse"
        n240 = event-data() -> ()  [unwired: 1 in, 1 out]
        n241 = property on="Command Selection" class="MCListbox (strict)"() -> ("ItemNames"=w395:string[][])  [unwired: 2 in, 2 out]
        n242 = Index Array(array=w395, index (row)="Command Selection", index (col)=0) -> (element=w393:string)
        n243 = call <vilib>:"Invoke Commands.vi"("Command Params"="Command Params", "Function Name"=w393) -> ("Params"=w389:u8, "Started"=w388:bool)  [unwired: 7 in, 1 out]
        n244 = Array Subset(array="Command Params", length (row)=w389) -> (w390:string[][])  [unwired: 3 in]
        n245 = Select(t="Executing" ("Cmd Status"), s=w388, f="" ("Cmd Status")) -> (s? t:f=→"Cmd Status":string)
      }
      event "Command Selection": Double Click {
        n246 = event-data() -> ("Row"=w403:i32)  [unwired: 1 in]
        n247 = property on="Command Selection" class="MCListbox (strict)"() -> ("ItemNames"=w406:string[][])  [unwired: 2 in, 2 out]
        n248 = local read "Command Params"() -> (w402:string[][])
        n249 = Index Array(array=w406, index (row)=w403, index (col)=0) -> (element=w404:string)
        n250 = call <vilib>:"Invoke Commands.vi"("Command Params"=w402, "Function Name"=w404) -> ("Params"=w401:u8, "Started"=w396:bool)  [unwired: 7 in, 1 out]
        n251 = Array Subset(array=w402, length (row)=w401) -> (w400:string[][])  [unwired: 3 in]
        n252 = Select(t="Executing" ("Cmd Status"), s=w396, f="" ("Cmd Status")) -> (s? t:f=w397:string)
        n253 = local write "Cmd Status"(w397) -> ()
      }
      event "CheckList": Double Click {
        # "Shift clears all"
        # "Update symbols on the listbox"
        n254 = event-data() -> ("PlatMods.Shift"=w408:bool, "Row"=w410:i32)  [unwired: 1 in]
        n255 = case shown="True" w408 {
          tunnel: w410 -> [w414 _]
          tunnel: 1 -> [w413 _]
          frame False {
            n256 = property on="CheckList" class="LstBox (strict)"() -> ("Item Symbols"=w412:i32[])  [unwired: 2 in, 2 out]
            n257 = Replace Array Subset(array=w412, new element=w413, index=w414) -> (w411:i32[])
            n258 = property on="CheckList" class="LstBox (strict)"("Item Symbols"=w411) -> ()  [unwired: 2 in, 2 out]
          }
          frame True {
            w415 = 0 ("Top Row")
            n259 = property on="CheckList" class="LstBox (strict)"() -> ("Number of Rows"=w417:u32)  [unwired: 2 in, 2 out]
            n260 = Initialize Array(0, w417) -> (w416:i32[])
            n261 = property on="CheckList" class="LstBox (strict)"("Top Row"=w415, "Value"=w415, "Item Symbols"=w416) -> ()  [unwired: 2 in, 2 out]
          }
        }
      }
      event "CheckList": Key Down {
        # "Update symbols on the listbox\nLeft and right keys check and uncheck"
        n262 = event-data() -> ("VKey"=w421:T19)  [unwired: 1 in]
        n263 = case shown="\"Left\", \"Right\"" w421 {
          selector: w421 -> [w426 _]
          tunnel: eventvkey."Left" ("VKey") -> [w424 _]
          frame "Left", "Right" {
            n264 = Equal?(x=w424, y=w426) -> (x = y?=w425:bool)
            n265 = Select(t=0, s=w425, f=1) -> (s? t:f=w427:i32)
            n266 = property on="CheckList" class="LstBox (strict)"() -> ("Item Symbols"=w430:i32[])  [unwired: 2 in, 2 out]
            n267 = Replace Array Subset(array=w430, new element=w427, index="CheckList") -> (w429:i32[])
            n268 = property on="CheckList" class="LstBox (strict)"("Item Symbols"=w429) -> ()  [unwired: 2 in, 2 out]
          }
          frame Default {
          }
        }
      }
      event "Motor.Enable": Value Change {
        # "When the test mode otor enable helper is set, update that\ntree row item's value"
        n269 = event-data() -> ("NewVal"=w436:bool)  [unwired: 1 in]
        n270 = Unbundle("Motor") -> ("Value"=w435:dbl)  [unwired: 1 out]
        n271 = Select(t=w435, s=w436, f=0.0) -> (s? t:f=w433:dbl)
        n272 = call <vilib>:"NT Write Number.vi"("Numeric"=w433, "Name"=w432) -> ()  [unwired: 9 in, 1 out]
      }
      event "Test Slider": Value Change {
        # "When the test mode slider helper is set, update that\ntree row item's value"
        n273 = event-data() -> ("NewVal"=w439:dbl)  [unwired: 1 in]
        n274 = call <vilib>:"NT Write Number.vi"("Numeric"=w439, "Name"=w440) -> ()  [unwired: 9 in, 1 out]
      }
      event "On/Off": Value Change {
        # "When the test mode on/off helper value is set, update that\ntree row item's value"
        n275 = event-data() -> ("NewVal"=w444:bool)  [unwired: 1 in]
        n276 = Boolean To (0,1)(Boolean=w444) -> (0, 1=w443:i16)
        n277 = call <vilib>:"NT Write Number.vi"("Numeric"=w443, "Name"=w442) -> ()  [unwired: 9 in, 1 out]
      }
      event "Rev/Fwd": Value Change {
        # "When the test mode helper value for relays is set, update that\ntree row item's value"
        n278 = event-data() -> ("NewVal.Forward"=w452:bool, "NewVal.Reverse"=w451:bool)  [unwired: 1 in]
        n279 = Boolean To (0,1)(Boolean=w452) -> (0, 1=w448:i16)
        n280 = Boolean To (0,1)(Boolean=w451) -> (0, 1=w450:i16)
        n281 = Negate(x=w450) -> (-x=w449:i16)
        n282 = Add(x=w448, y=w449) -> (x+y=w447:i16)
        n283 = call <vilib>:"NT Write Number.vi"("Numeric"=w447, "Name"=w446) -> ()  [unwired: 9 in, 1 out]
      }
      event "Test Ring": Value Change {
        # "When a test mode helper value is selected from the ring,\nset the tree item's variable to the string value"
        n284 = event-data() -> ("NewVal"=w456:u16)  [unwired: 1 in]
        n285 = property on="Test Ring" class="Ring (strict)"() -> ("Strings []"=w457:string[])  [unwired: 2 in, 2 out]
        n286 = Index Array(array=w457, index=w456) -> (element=w455:string)
        n287 = call <vilib>:"NT Write String.vi"("String"=w455, "Name"=w454) -> ()  [unwired: 9 in, 1 out]
      }
      event "Rec Mode": Value Change {
        # "Update globals for recording mode and path to read log from.\nClear when logging and let NetworkTables set path for vision to\nuse."
        n288 = event-data() -> ("NewVal"=w468:enum32{"Stop", "Record", "Playback"})  [unwired: 1 in]
        n289 = global write "WPI_DashboardLogging Global.vi" "Logging Filename"(path "") -> ()
        n290 = global write "WPI_DashboardLogging Global.vi" "Recording"(w468) -> ()
        n291 = case shown="\"Playback\"" w468 {
          tunnel: w467 -> [_ w470 w479]
          tunnel: [_ _ w478] -> w465
          tunnel: [_ _ w477] -> _
          tunnel: w463 -> [_ _ w475]
          tunnel: cluster{i32, i32} {-250, 170} -> [_ _ w474]
          tunnel: [_ _ T20 {"Image Size"=TRUE, "Image Type"=TRUE, "Pixel Value"=TRUE, "ROI Information"=TRUE, "Zoom Factor"=FALSE} ("Image Information Shown:All Elements")] -> w461
          tunnel: [_ _ TRUE ("Zoom Factor")] -> w460
          tunnel: w459 -> [_ _ w471]
          frame Default {
          }
          frame "Stop", "Record" {
            # "Place Window too"
            n292 = invoke class="VI" method="FP.Close"(reference=w470) -> (reference out=w469:refnum<vi>)  [unwired: 2 in, 2 out]
            n293 = invoke class="VI" method="Abort VI"(reference=w469) -> ()  [unwired: 2 in, 3 out]
          }
          frame "Playback" {
            n294 = call "Open Playback Panel.vi"("Offset"=w474, "DB VI Ref"=w475, "Playback in"=w479) -> ("Playback out"=w476:refnum<vi>)  [unwired: 8 in]
            n295 = register-events(w476, w471) -> (reference out=w478:refnum<event-registration>, error out=w477:errorcluster)  [unwired: 2 in]
          }
        }
        n296 = property on="Camera Image" class="ImageControl"("Image Information Shown"=w461, "Image Information Visible"=w460) -> ()  [unwired: 2 in, 2 out]
        n297 = call <vilib>:"WPI_DashboardNT Log FieldName Cache.vi"("Operation"=enum16{"Lookup/Add", "Index", "Clear"}."Clear") -> ()  [unwired: 8 in, 3 out]
      }
      event Panel Close {
        w481 = enum32{"Stop", "Record", "Playback"}."Stop" ("Rec Mode")
        # "Playback window has been closed, abort"
        n298 = event-data() -> ()  [unwired: 1 in, 4 out]
        n299 = local write "Rec Mode"(w481) -> ()
        n300 = global write "WPI_DashboardLogging Global.vi" "Recording"(w481) -> ()
      }
      event Panel Close {
        # "Abort playback window and ourself"
        n301 = event-data() -> ()  [unwired: 1 in, 4 out]
        n302 = invoke class="VI" method="FP.Close"(reference=w485) -> (reference out=w484:refnum<vi>)  [unwired: 2 in, 2 out]
        n303 = invoke class="VI" method="Abort VI"(reference=w484) -> (error out=w483:errorcluster)  [unwired: 2 in, 2 out]
        n304 = invoke class="VI" method="Abort VI"(error in=w483) -> ()  [unwired: 2 in, 3 out]
      }
      event User Event {
        n305 = event-data() -> ("IDs"=w492:cluster{"RPC field ID":u16, "Unique ID":u16}, "String"=w491:string)  [unwired: 1 in]
        n306 = Bundle("IDs"=w492, "String"=w491) -> (w490:T8)  [unwired: 1 in]
        n307 = call <vilib>:"Retrieve RPC Response.vi"("RPC Response"=w490) -> ("Output"=w488:string[][])  [unwired: 10 in]
        n308 = Build Array (concatenate)(w486, w488) -> (w487:string[][])
        n309 = local write "Command Params"(w487) -> ()
        n310 = local write "Cmd Status"("" ("Cmd Status")) -> ()
      }
      event "Tree": Double Click {
        n311 = event-data() -> ("PlatMods"=w496:T23, "Tag"=w495:string)  [unwired: 1 in]
        n312 = Unbundle(w496) -> ("Shift"=w494:bool)  [unwired: 4 out]
        n313 = Not(x=w494) -> (.not. x?=w493:bool)
        n314 = call <vilib>:"NT Update Persistence.vi"("Persistence"=w493, "Name"=w495) -> ()  [unwired: 9 in, 1 out]
      }
    }
  }
  n315 = while {
    tunnel: w81 -> [w499]
    i -> [w502]
    stop <- FALSE stop-if-true
    n316 = Wait (ms)(milliseconds to wait=u32 100) -> ()  [unwired: 1 out]
    n317 = case shown="\"Playback\"" "Rec Mode" {
      tunnel: w502 -> [_ _ w517]
      tunnel: [u32 2829099 ("Base Color") u32 11141120 ("Target Color") w506] -> w498
      frame "Stop", Default {
        # "Reset the color, extra updates don't cost much"
      }
      frame "Record" {
      }
      frame "Playback" {
        # "Playback"
        n318 = Quotient & Remainder(x=w517, y=u32 50 ("milliseconds to wait")) -> (x-y*floor(x/y)=w513:u32)  [unwired: 1 out]
        n319 = Divide(x=w513, y=u32 50 ("milliseconds to wait")) -> (x/y=w510:dbl)
        n320 = Multiply(x=6.283185307179586, y=w510) -> (x*y=w515:dbl)
        n321 = Sine(x=w515) -> (sin(x)=w514:dbl)
        n322 = Absolute Value(x=w514) -> (abs(x)=w507:dbl)
        n323 = call "Interpolate RGB Color.vi"("Proportion"=w507, "Target Color"=u32 30976, "Base Color"=u32 2829099) -> ("Result Color"=w506:u32)  [unwired: 8 in]
      }
    }
    n324 = property class="Pane"(reference=w499, "PaneColor"=w498) -> ()  [unwired: 1 in, 2 out]
  }
  n325 = local write "Dashboard Tab"(T2."Drive" ("Dashboard Tab")) -> ()
  n326 = property on="On/Off" class="Bool (strict)"("Visible"=w50) -> ()  [unwired: 2 in, 2 out]
  n327 = property on="Motor" class="Clust (strict)"("Visible"=w50) -> ()  [unwired: 2 in, 2 out]
  n328 = property on="Progress" class="Clust (strict)"("Visible"=w50) -> ()  [unwired: 2 in, 2 out]
  n329 = property on="Test Ring" class="Ring (strict)"("Visible"=w50) -> ()  [unwired: 2 in, 2 out]
  n330 = property on="Rev/Fwd" class="Clust (strict)"("Visible"=w50) -> ()  [unwired: 2 in, 2 out]
  n331 = while {
    tunnel: u16 1741 ("timeout ms (25000)") -> [w519]
    stop <- FALSE stop-if-true
    n332 = TCP Create Listener(10:w519) -> (0:w518:errorcluster, 3:w520:refnum<k5>)  [unwired: 4 in, 1 out]
    n333 = case shown="No Error" w518 {
      selector: w518 -> [w522 _]
      tunnel: w520 -> [w523 _]
      frame No Error {
        n334 = while {
          tunnel: w523 -> [w526]
          tunnel: w522 -> [w525]
          stop <- FALSE stop-if-true
          n335 = TCP Wait On Listener(8:w525, 11:w526) -> (0:w527:errorcluster, 4:w528:refnum<k5>)  [unwired: 2 in, 3 out]
          n336 = local write "TCP"(w528) -> ()
          n337 = case shown="No Error" w527 {
            frame No Error {
            }
            frame Error {
              n338 = Wait (ms)(milliseconds to wait=u32 1000) -> ()  [unwired: 1 out]
            }
          }
        }
      }
      frame Error {
        n339 = Wait (ms)(milliseconds to wait=u32 1000) -> ()  [unwired: 1 out]
      }
    }
  }
  n340 = local write "Command Selection"(u16 0 ("milliseconds to wait")) -> ()
  n341 = local write "Command Params"(string[][] [] ("Command Params")) -> ()
  n342 = global write "WPI_DashboardLogging Global.vi" "Recording"(w75) -> ()
  n343 = local write "Rec Mode"(w75) -> ()
  n344 = call <vilib>:"NT Write String.vi"("String"="Select Auto", "Name"="Auto Selector") -> ()  [unwired: 9 in, 1 out]
